vi "myRIO_BRig_RT_dataMTrig_Solenoid_delay__L.vi"() -> (2 "output_Solenoid_delay__L":i32)   [LabVIEW 2014]
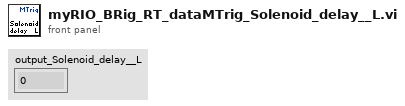
[diagram p1: front panel]
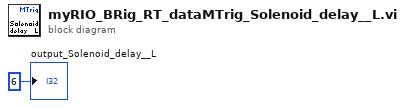
[diagram p0: block diagram]
diagram:
  "output_Solenoid_delay__L" <- 6 ("output_iBlock")
